vi "Write Device.vi"(8 "error in (no error)":errorcluster, 10 "Device":i32, 11 "Launch Hardware Settings Msg in":refnum<class "Launch Hardware Settings Msg.lvclass">) -> (0 "error out":errorcluster, 3 "Launch Hardware Settings Msg out":refnum<class "Launch Hardware Settings Msg.lvclass">)   [LabVIEW 2016, in "Measurement UI.lvlib" / "Launch Hardware Settings Msg.lvclass"]
uses:
  Launch Hardware Settings Msg.lvclass
  Launch Hardware Settings Msg.lvclass/Launch Hardware Settings Msg.ctl
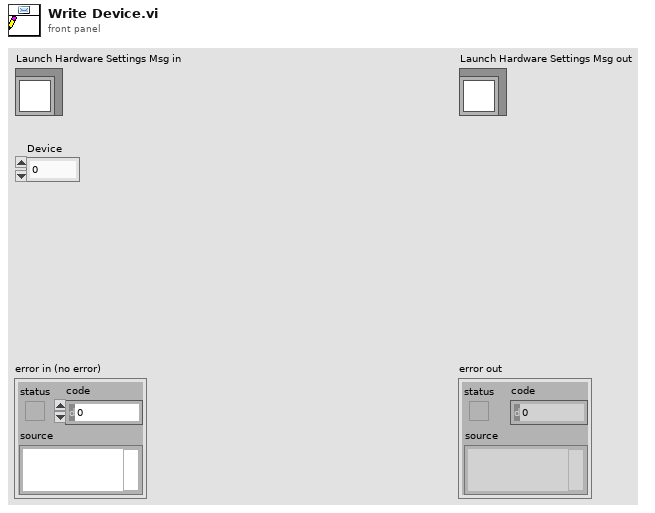
[diagram p1: front panel]
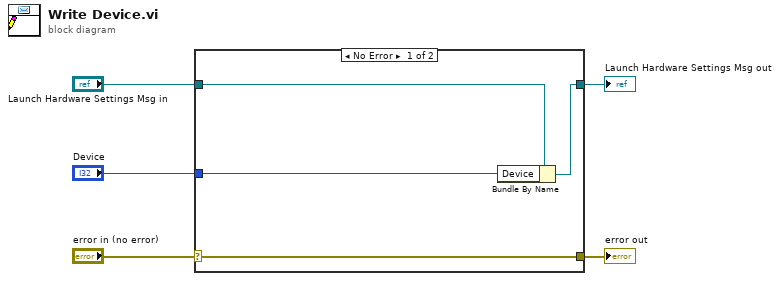
[diagram p0: block diagram]
diagram:
  n1 = case shown="No Error" "error in (no error)" {
    selector: "error in (no error)" -> [w9 w10]
    tunnel: [w9 w10] -> w4
    tunnel: [w7 w11] -> w2
    tunnel: "Launch Hardware Settings Msg in" -> [w8 w11]
    tunnel: "Device" -> [w6 _]
    frame No Error {
      n2 = Bundle By Name(cluster=w8, "Device"=w6) -> (w7:refnum<class "Launch Hardware Settings Msg.lvclass">)
    }
    frame Error {
    }
  }
  "error out" <- w4
  "Launch Hardware Settings Msg out" <- w2
